vi "Read Voltage Measurement.vi"   [LabVIEW 2013, in "Cal Inst.lvlib" / "California Instruments iX Series.lvlib"]
doc: "Reads single of multiple voltage measurement(s)."
uses:
  California Instruments iX Series.lvlib
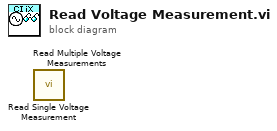
[diagram p0: block diagram]
diagram:
  n1 = call "Read Single Voltage Measurement.vi"() -> ()  [unwired: 9 in, 3 out]
  n2 = call "Read Multiple Voltage Measurements.vi"() -> ()  [unwired: 9 in, 3 out]
